vi "Square Wave Generator LUT.vi"(0 "frequency (periods/tick)":fxp<+,32,0>=0.0002500000409781933, 1 "reset":bool, 5 "phase offset (periods)":fxp<+,32,0>) -> (4 "saw out":i16)   [LabVIEW 2015]
doc: "Generates a point-by-point triangle wave using direct digital synthesis. The synthesis runs continuously from the top-level FPGA target clock to produce an accurate real-time frequency. Each execution of this VI returns the most recent sample produced by the underlying synthesis engine."
uses:
  <vilib>/rvi/Analysis/common/FxpNativeNode/niFpgaFxpNative.xnode
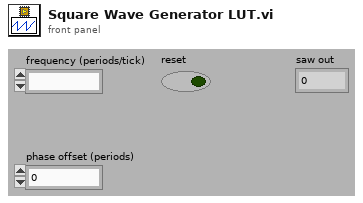
[diagram p1: front panel]
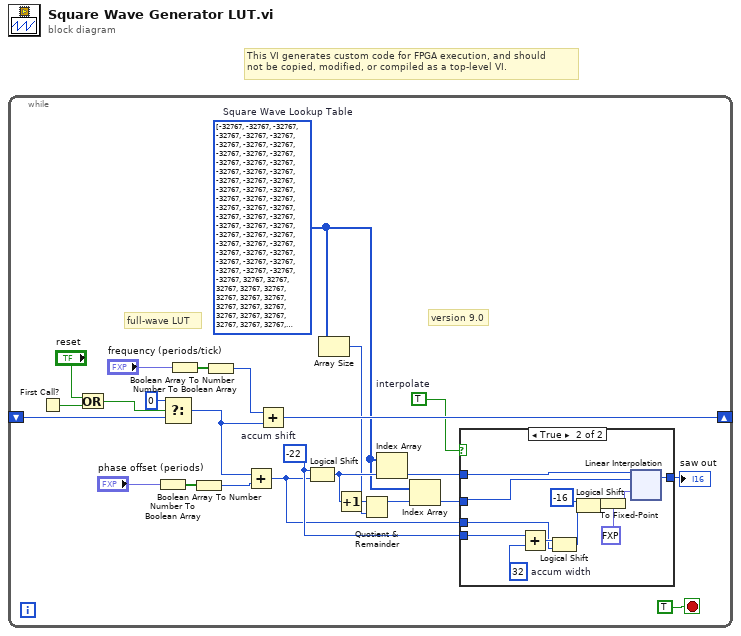
[diagram p0: block diagram]
diagram:
  # "This VI generates custom code for FPGA execution, and should\nnot be copied, modified, or compiled as a top-level VI."
  n1 = while {
    shift-right: [w24] -> _
    shift-left: _ -> [w17]
    stop <- TRUE stop-if-true
    w1 = i16[] [-32767, -32767, -32767, -32767, -32767, -32767, -32767, -32767, -32767, -32767, -32767, -32767, -32767, -32767, -32767, -32767, -32767, -32767, -32767, -32767, -32767, -32767, -32767, -32767, -32767, -32767, -32767, -32767, -32767, -32767, -32767, -32767, -32767, -32767, -32767, -32767, -32767, -32767, -32767, -32767, -32767, -32767, -32767, -32767, -32767, -32767, -32767, -32767, -32767, -32767, -32767, -32767, 32767, 32767, 32767, 32767, 32767, 32767, 32767, 32767, 32767, 32767, 32767, 32767, 32767, 32767, 32767, 32767, 32767, 32767, 32767, 32767, 32767, 32767, 32767, 32767, 32767, 32767, 32767, 32767, 32767, 32767, 32767, 32767, 32767, 32767, 32767, 32767, 32767, 32767, 32767, 32767, 32767, 32767, 32767, 32767, 32767, 32767, 32767, 32767, 32767, 32767, 32767, -32767, -32767, -32767, -32767, -32767, -32767, -32767, -32767, -32767, -32767, -32767, -32767, -32767, -32767, -32767, -32767, -32767, -32767, -32767, -32767, -32767, -32767, -32767, -32767, -32767, -32767, -32767, -32767, -32767, -32767, -32767, -32767, -32767, -32767, -32767, -32767, -32767, -32767, -32767, -32767, -32767, -32767, -32767, -32767, -32767, -32767, -32767, -32767, -32767, -32767, -32767, 32767, 32767, 32767, 32767, 32767, 32767, 32767, 32767, 32767, 32767, 32767, 32767, 32767, 32767, 32767, 32767, 32767, 32767, 32767, 32767, 32767, 32767, 32767, 32767, 32767, 32767, 32767, 32767, 32767, 32767, 32767, 32767, 32767, 32767, 32767, 32767, 32767, 32767, 32767, 32767, 32767, 32767, 32767, 32767, 32767, 32767, 32767, 32767, 32767, 32767, 32767, -32767, -32767, -32767, -32767, -32767, -32767, -32767, -32767, -32767, -32767, -32767, -32767, -32767, -32767, -32767, -32767, -32767, -32767, -32767, -32767, -32767, -32767, -32767, -32767, -32767, -32767, -32767, -32767, -32767, -32767, -32767, -32767, -32767, -32767, -32767, -32767, -32767, -32767, -32767, -32767, -32767, -32767, -32767, -32767, -32767, -32767, -32767, -32767, -32767, -32767, -32767, 32767, 32767, 32767, 32767, 32767, 32767, 32767, 32767, 32767, 32767, 32767, 32767, 32767, 32767, 32767, 32767, 32767, 32767, 32767, 32767, 32767, 32767, 32767, 32767, 32767, 32767, 32767, 32767, 32767, 32767, 32767, 32767, 32767, 32767, 32767, 32767, 32767, 32767, 32767, 32767, 32767, 32767, 32767, 32767, 32767, 32767, 32767, 32767, 32767, 32767, 32767, 32767, -32767, -32767, -32767, -32767, -32767, -32767, -32767, -32767, -32767, -32767, -32767, -32767, -32767, -32767, -32767, -32767, -32767, -32767, -32767, -32767, -32767, -32767, -32767, -32767, -32767, -32767, -32767, -32767, -32767, -32767, -32767, -32767, -32767, -32767, -32767, -32767, -32767, -32767, -32767, -32767, -32767, -32767, -32767, -32767, -32767, -32767, -32767, -32767, -32767, -32767, -32767, 32767, 32767, 32767, 32767, 32767, 32767, 32767, 32767, 32767, 32767, 32767, 32767, 32767, 32767, 32767, 32767, 32767, 32767, 32767, 32767, 32767, 32767, 32767, 32767, 32767, 32767, 32767, 32767, 32767, 32767, 32767, 32767, 32767, 32767, 32767, 32767, 32767, 32767, 32767, 32767, 32767, 32767, 32767, 32767, 32767, 32767, 32767, 32767, 32767, 32767, 32767, -32767, -32767, -32767, -32767, -32767, -32767, -32767, -32767, -32767, -32767, -32767, -32767, -32767, -32767, -32767, -32767, -32767, -32767, -32767, -32767, -32767, -32767, -32767, -32767, -32767, -32767, -32767, -32767, -32767, -32767, -32767, -32767, -32767, -32767, -32767, -32767, -32767, -32767, -32767, -32767, -32767, -32767, -32767, -32767, -32767, -32767, -32767, -32767, -32767, -32767, -32767, 32767, 32767, 32767, 32767, 32767, 32767, 32767, 32767, 32767, 32767, 32767, 32767, 32767, 32767, 32767, 32767, 32767, 32767, 32767, 32767, 32767, 32767, 32767, 32767, 32767, 32767, 32767, 32767, 32767, 32767, 32767, 32767, 32767, 32767, 32767, 32767, 32767, 32767, 32767, 32767, 32767, 32767, 32767, 32767, 32767, 32767, 32767, 32767, 32767, 32767, 32767, -32767, -32767, -32767, -32767, -32767, -32767, -32767, -32767, -32767, -32767, -32767, -32767, -32767, -32767, -32767, -32767, -32767, -32767, -32767, -32767, -32767, -32767, -32767, -32767, -32767, -32767, -32767, -32767, -32767, -32767, -32767, -32767, -32767, -32767, -32767, -32767, -32767, -32767, -32767, -32767, -32767, -32767, -32767, -32767, -32767, -32767, -32767, -32767, -32767, -32767, -32767, -32767, 32767, 32767, 32767, 32767, 32767, 32767, 32767, 32767, 32767, 32767, 32767, 32767, 32767, 32767, 32767, 32767, 32767, 32767, 32767, 32767, 32767, 32767, 32767, 32767, 32767, 32767, 32767, 32767, 32767, 32767, 32767, 32767, 32767, 32767, 32767, 32767, 32767, 32767, 32767, 32767, 32767, 32767, 32767, 32767, 32767, 32767, 32767, 32767, 32767, 32767, 32767, -32767, -32767, -32767, -32767, -32767, -32767, -32767, -32767, -32767, -32767, -32767, -32767, -32767, -32767, -32767, -32767, -32767, -32767, -32767, -32767, -32767, -32767, -32767, -32767, -32767, -32767, -32767, -32767, -32767, -32767, -32767, -32767, -32767, -32767, -32767, -32767, -32767, -32767, -32767, -32767, -32767, -32767, -32767, -32767, -32767, -32767, -32767, -32767, -32767, -32767, -32767, 32767, 32767, 32767, 32767, 32767, 32767, 32767, 32767, 32767, 32767, 32767, 32767, 32767, 32767, 32767, 32767, 32767, 32767, 32767, 32767, 32767, 32767, 32767, 32767, 32767, 32767, 32767, 32767, 32767, 32767, 32767, 32767, 32767, 32767, 32767, 32767, 32767, 32767, 32767, 32767, 32767, 32767, 32767, 32767, 32767, 32767, 32767, 32767, 32767, 32767, 32767, -32767, -32767, -32767, -32767, -32767, -32767, -32767, -32767, -32767, -32767, -32767, -32767, -32767, -32767, -32767, -32767, -32767, -32767, -32767, -32767, -32767, -32767, -32767, -32767, -32767, -32767, -32767, -32767, -32767, -32767, -32767, -32767, -32767, -32767, -32767, -32767, -32767, -32767, -32767, -32767, -32767, -32767, -32767, -32767, -32767, -32767, -32767, -32767, -32767, -32767, -32767, 32767, 32767, 32767, 32767, 32767, 32767, 32767, 32767, 32767, 32767, 32767, 32767, 32767, 32767, 32767, 32767, 32767, 32767, 32767, 32767, 32767, 32767, 32767, 32767, 32767, 32767, 32767, 32767, 32767, 32767, 32767, 32767, 32767, 32767, 32767, 32767, 32767, 32767, 32767, 32767, 32767, 32767, 32767, 32767, 32767, 32767, 32767, 32767, 32767, 32767, 32767, 32767, -32767, -32767, -32767, -32767, -32767, -32767, -32767, -32767, -32767, -32767, -32767, -32767, -32767, -32767, -32767, -32767, -32767, -32767, -32767, -32767, -32767, -32767, -32767, -32767, -32767, -32767, -32767, -32767, -32767, -32767, -32767, -32767, -32767, -32767, -32767, -32767, -32767, -32767, -32767, -32767, -32767, -32767, -32767, -32767, -32767, -32767, -32767, -32767, -32767, -32767, -32767, 32767, 32767, 32767, 32767, 32767, 32767, 32767, 32767, 32767, 32767, 32767, 32767, 32767, 32767, 32767, 32767, 32767, 32767, 32767, 32767, 32767, 32767, 32767, 32767, 32767, 32767, 32767, 32767, 32767, 32767, 32767, 32767, 32767, 32767, 32767, 32767, 32767, 32767, 32767, 32767, 32767, 32767, 32767, 32767, 32767, 32767, 32767, 32767, 32767, 32767, 32767, -32767, -32767, -32767, -32767, -32767, -32767, -32767, -32767, -32767, -32767, -32767, -32767, -32767, -32767, -32767, -32767, -32767, -32767, -32767, -32767, -32767, -32767, -32767, -32767, -32767, -32767, -32767, -32767, -32767, -32767, -32767, -32767, -32767, -32767, -32767, -32767, -32767, -32767, -32767, -32767, -32767, -32767, -32767, -32767, -32767, -32767, -32767, -32767, -32767, -32767, -32767, 32767, 32767, 32767, 32767, 32767, 32767, 32767, 32767, 32767, 32767, 32767, 32767, 32767, 32767, 32767, 32767, 32767, 32767, 32767, 32767, 32767, 32767, 32767, 32767, 32767, 32767, 32767, 32767, 32767, 32767, 32767, 32767, 32767, 32767, 32767, 32767, 32767, 32767, 32767, 32767, 32767, 32767, 32767, 32767, 32767, 32767, 32767, 32767, 32767, 32767, 32767]  # Square Wave Lookup Table
    w20 = TRUE  # interpolate
    w19 = i8 -22  # accum shift
    # "version 9.0"
    # "full-wave LUT"
    n2 = First Call?() -> (First Call?: T/F=w15:bool)
    n3 = Or(x="reset", y=w15) -> (x .or. y?=w14:bool)
    n4 = Number To Boolean Array(number="phase offset (periods)") -> (Boolean array=w4:bool[])
    n5 = Select(t=u32 0, s=w14, f=w17) -> (s? t:f=w22:u32)
    n6 = Number To Boolean Array(number="frequency (periods/tick)") -> (Boolean array=w7:bool[])
    n7 = Boolean Array To Number(Boolean array=w4) -> (number=w2:u32)
    n8 = Boolean Array To Number(Boolean array=w7) -> (number=w5:u32)
    n9 = Add(x=w22, y=w2) -> (x+y=w18:u32)
    n10 = Add(x=w5, y=w22) -> (x+y=w24:u32)
    n11 = Logical Shift(y=w19, x=w18) -> (x << y=w12:u32)
    n12 = Array Size(array=w1) -> (size(s)=w8:i32)
    n13 = Increment(x=w12) -> (x+1=w13:u32)
    n14 = Quotient & Remainder(x=w13, y=w8) -> (x-y*floor(x/y)=w10:u32)  [unwired: 1 out]
    n15 = Index Array(array=w1, index=w12) -> (element=w11:i16)
    n16 = Index Array(array=w1, index=w10) -> (element=w9:i16)
    n17 = case shown="True" w20 {
      tunnel: w11 -> [w26 w29]
      tunnel: [w26 w28] -> w21
      tunnel: w19 -> [_ w38]
      tunnel: w18 -> [_ w35]
      tunnel: w9 -> [_ w30]
      frame False {
      }
      frame True {
        w37 = i8 32  # accum width
        n18 = Add(x=w38, y=w37) -> (x+y=w36:i8)
        n19 = Logical Shift(y=w36, x=w35) -> (x << y=w34:u32)
        n20 = Logical Shift(y=-16, x=w34) -> (x << y=w32:u32)
        n21 = To Fixed-Point(fixed-point type=fxp<+,16,0> 0.0, number=w32) -> (fixed-point=w31:fxp<+,16,0>)
        n22 = xnode ("Linear Interpolation")("y0"=w29, "y1"=w30, "x"=w31) -> ("y"=w28:i16)
      }
    }
    "saw out" <- w21
  }
